vi "frontPanels.vi"() -> ()   [LabVIEW 2020]
uses:
  C:/Users/DESKTOP-TLO0G68A/Desktop/LabVIEW/instrumentationLV/Thorlabs.MotionControl.Controls.dll
  Thorlabs.MotionControl.Controls.dll
  C:/Users/DESKTOP-TLO0G68A/Desktop/LabVIEW/instrumentationLV/ThorLabs.MotionControl.KCube.DCServoCLI.dll
  ThorLabs.MotionControl.KCube.DCServoCLI.dll
  C:/Users/DESKTOP-TLO0G68A/Desktop/LabVIEW/instrumentationLV/Thorlabs.MotionControl.GenericMotorCLI.dll
  Thorlabs.MotionControl.GenericMotorCLI.dll
panel:
  in  "Begin Scan":bool
  in  "SerialNumber":string="27502753"
  in  "KCubeDCServoControl":refnum<k24>(container)
  in  "x steps":dbl=5.0
  in  "step size":dbl=1.0
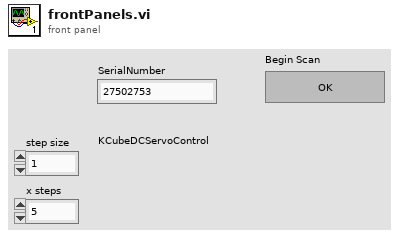
[diagram p1: front panel]
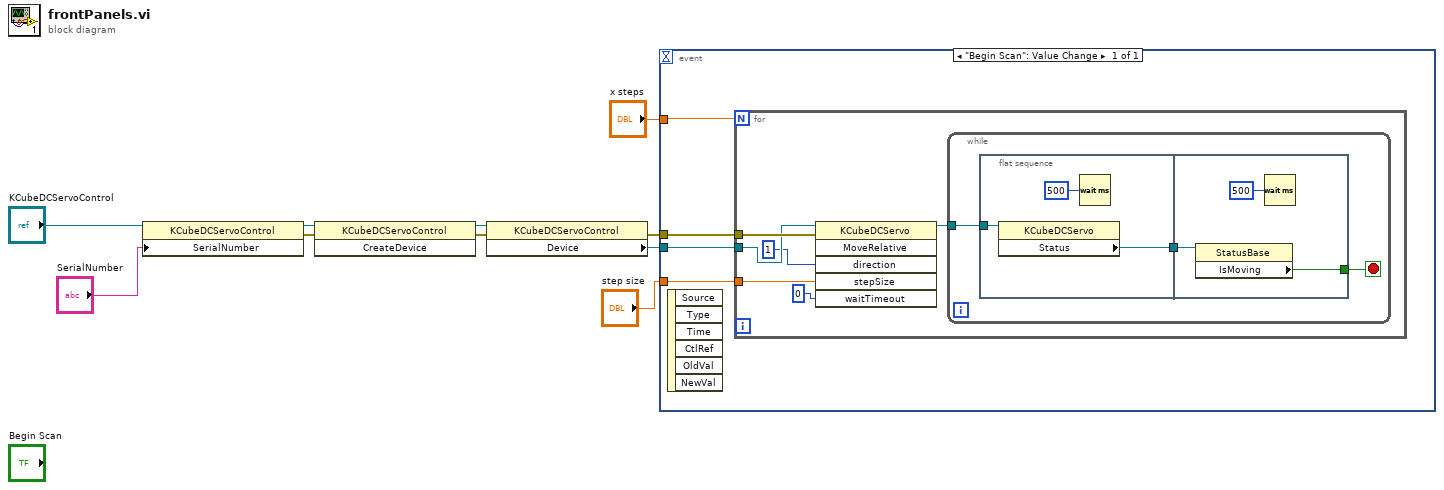
[diagram p0: block diagram]
diagram:
  n1 = property class="KCubeDCServoControl"(reference="KCubeDCServoControl", "SerialNumber"="SerialNumber") -> (reference out=w9:refnum<k24>, error out=w7:errorcluster)  [unwired: 1 in]
  n2 = invoke class="KCubeDCServoControl" method="CreateDevice"(reference=w9, error in=w7) -> (reference out=w8:refnum<k24>, error out=w6:errorcluster)  [unwired: 1 in, 1 out]
  n3 = property class="KCubeDCServoControl"(reference=w8, error in=w6) -> (error out=w3:errorcluster, "Device"=w4:refnum<k24>)  [unwired: 1 out]
  n4 = event shown="[0] \"Begin Scan\": Value Change" {
    selector: _ -> [_]
    dyn-events: _ -> [_]
    timeout: _ -> [_]
    tunnel: w4 -> [w14]
    tunnel: w3 -> [w13]
    tunnel: "step size" -> [w12]
    tunnel: "x steps" -> [w11]
    event "Begin Scan": Value Change {
      n5 = event-data() -> ()  [unwired: 1 in, 6 out]
      n6 = for {
        N: w11 -> [_]
        tunnel: w14 -> [w18]
        tunnel: w13 -> [w20]
        tunnel: w12 -> [w19]
        n7 = invoke class="KCubeDCServo" method="MoveRelative"(reference=w18, error in=w20, "direction"=1 ("waitTimeout"), "stepSize"=w19, "waitTimeout"=0) -> (reference out=w15:refnum<k24>)  [unwired: 1 in, 5 out]
        n8 = while {
          tunnel: w15 -> [w23]
          stop <- w22 stop-if-true
          n9 = flat-sequence {
            tunnel: w23 -> [w26]
            tunnel: [w25] -> w21
            tunnel: [w29] -> w22
            tunnel: w21 -> [w28]
            frame #0 {
              n10 = property class="KCubeDCServo"(reference=w26) -> ("Status"=w25:refnum<k24>)  [unwired: 1 in, 2 out]
              n11 = Wait (ms)(milliseconds to wait=500) -> ()  [unwired: 1 out]
            }
            frame #1 {
              n12 = property class="StatusBase"(reference=w28) -> ("IsMoving"=w29:bool)  [unwired: 1 in, 2 out]
              n13 = Wait (ms)(milliseconds to wait=500) -> ()  [unwired: 1 out]
            }
          }
        }
      }
    }
  }
